vi "byciclemobeltest.vi"() -> ()   [LabVIEW 2016]
uses:
  <vilib>/platform/TimedLoop/XDataNode/XDataNode.xnode
  <vilib>/Platform/TimedLoop/XDataNode/nitl_modes.ctl
  <vilib>/Platform/TimedLoop/XDataNode/XDNodeRunTimeDep.lvlib
  <vilib>/Platform/TimedLoop/XDataNode/wakeup.ctl
  <vilib>/Platform/TimedLoop/XDataNode/timing_clust.ctl
panel:
  out "New Vehicle Orientation Beta":dbl format="%.2f"
  in  "set runtime":u32
  in  "stop":bool
  out "XY Graph":cluster{dbl[], dbl[]}[](graph)
  in  "Wheel angle (deg)":dbl
  in  "Ground speed (km/h)":dbl
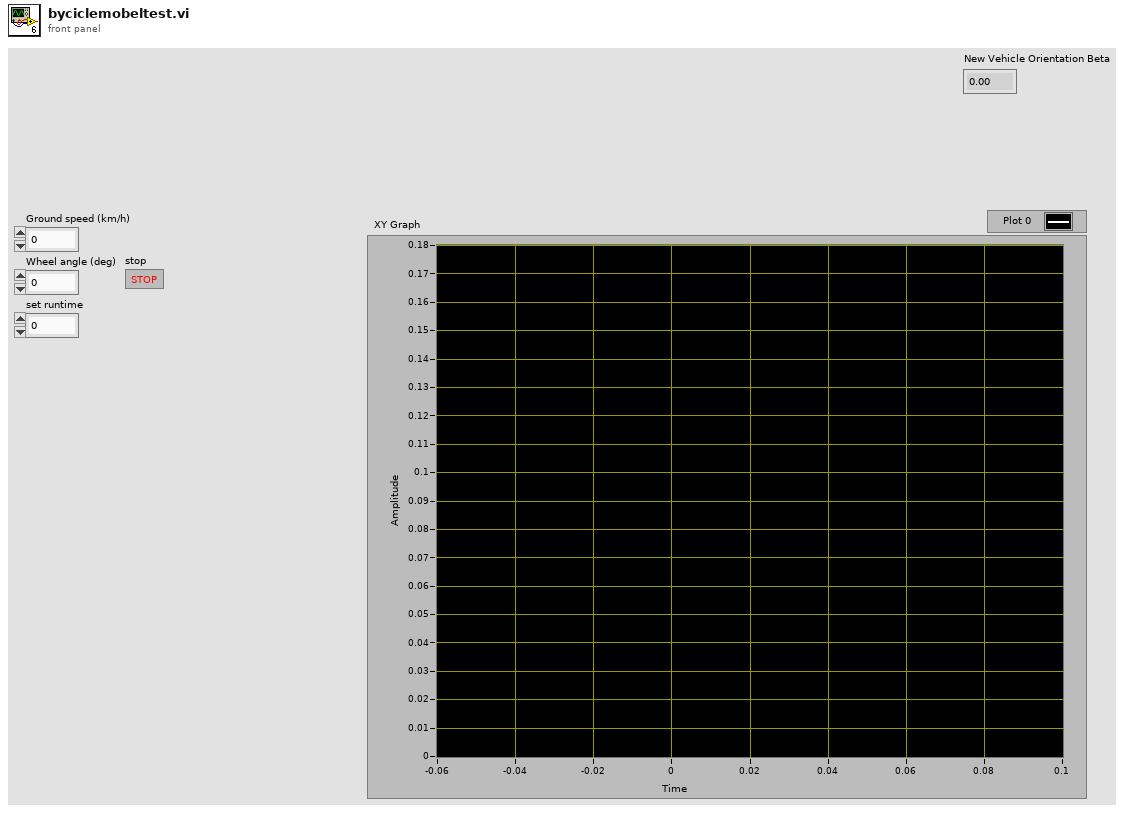
[diagram p1: front panel]
types:
  T1 = typedef "XDNodeRunTimeDep.lvlib/timing_clust.ctl" = cluster{"Expected End [f-1]":u64, "Actual End [f-1]":u64, "Finished Late? [f-1]":bool, "Expected End [i-1]":u64, "Actual End [i-1]":u64, "Finished Late? [i-1]":bool, "Expected Start [i]":u64, "Actual Start [i]":u64, "Expected Start [f]":u64, "Actual Start [f]":u64, "Source Name":string, "Structure Name":string, "Period":i64, "Deadline":i64, "Offset":i64, "Start":i64, "Priority":i32, "Timeout":i32, "Mode":T2, "Wakeup Reason":T3, "Error":errorcluster, "Source Type":string, "Secondary Source Type":string, "Global End Time":u64, "Global Start Time":u64, "Frame Duration":u64, "Iteration Duration":u64, "Assigned CPU":i32, "I/O Scan Engine Mode":u32}
  T2 = typedef "XDNodeRunTimeDep.lvlib/nitl_modes.ctl" = enum32{"No Change", "Process missed periods, maintain original phase", "Discard missed periods, maintain original phase", "Process missed periods, ignore original phase", "Discard missed periods, ignore original phase"}
  T3 = typedef "XDNodeRunTimeDep.lvlib/wakeup.ctl" = enum32{"Normal", "Aborted", "Asynchronous wakeup", "Timing source error", "Timed loop error", "Timeout"}
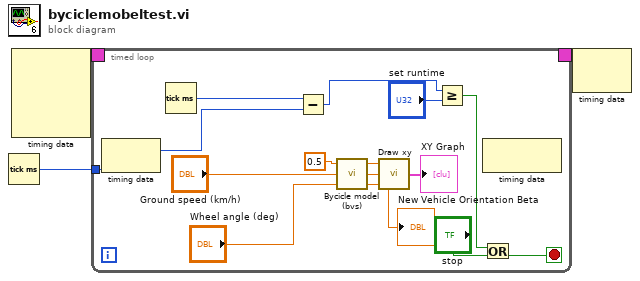
[diagram p0: block diagram]
diagram:
  n1 = Tick Count (ms)() -> (millisecond timer value=w1:u32)
  n2 = node-c288() -> (w3:T1)  [unwired: 4 in]
  n3 = timed-loop {
    timing: w3 -> [_]
    timing-out: [_] -> w2
    tunnel: w1 -> [w9]
    stop <- w6 stop-if-true
    n4 = node-c288() -> ()  [unwired: 1 in, 1 out]
    n5 = Tick Count (ms)() -> (millisecond timer value=w10:u32)
    n6 = Subtract(x=w10, y=w9) -> (x-y=w8:u32)
    n7 = call "Bycicle model (bvs).vi"("Wheel angle (deg)"="Wheel angle (deg)", "Ground speed (km/h)"="Ground speed (km/h)", "dt (s)"=0.5) -> ("New Vehicle Orientation Beta"=→"New Vehicle Orientation Beta":dbl, "New position Y"=w13:dbl, "New position X"=w14:dbl)
    n8 = call "Draw xy.vi"("Y"=w13, "x"=w14) -> ("XY Graph"=→"XY Graph":cluster{dbl[], dbl[]}[])  [unwired: 1 in]
    n9 = Greater Or Equal?(x=w8, y="set runtime") -> (x >= y?=w5:bool)
    n10 = node-c288() -> ()  [unwired: 1 in, 1 out]
    n11 = Or(x=w5, y="stop") -> (x .or. y?=w6:bool)
  }
  n12 = node-c288(w2) -> ()  [unwired: 1 out]
